vi "Run (lvsound2).vi"(8 "error in (no error)":errorcluster, 11 "Audio Output Queue":refnum<queue>) -> (0 "error out":errorcluster)   [LabVIEW 2019, in "Audio Output.lvlib"]
doc: "The main audio output loop.\n\n<b>Priority:</b> Time Critical\n<b>Execution System:</b> Instrument I/O"
uses:
  Audio Output.lvlib
  Audio Output Queue Type.ctl
  State.ctl
  Messaging/Message Cluster.ctl
  Audio Output Config.ctl
  Audio Output Info.ctl
  <vilib>/sound2/lvsound2.llb/Sound Data Format.ctl
  <vilib>/sound2/lvsound2.llb/Sound Output Task ID.ctl
  Globals/Constants.vi
  Globals/Debug.vi
  <vilib>/sound2/lvsound2.llb/Sound Output Write (I16).vi
  Messaging/Messaging.lvlib
  Globals/Globals.lvlib
  <vilib>/ptbypt/NI_PtbyPt.lvlib
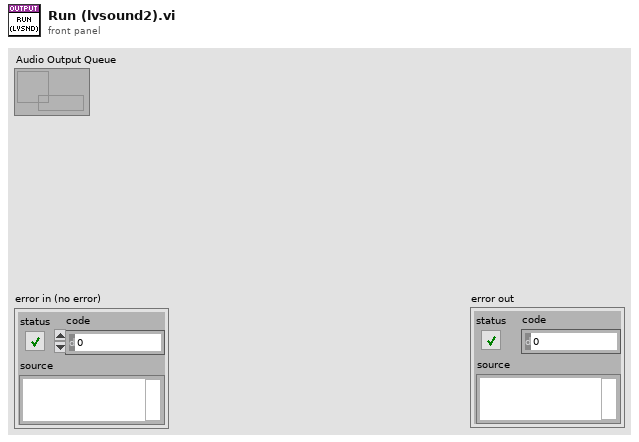
[diagram p1: front panel]
types:
  T1 = typedef "Audio Output.lvlib/Audio Output Config.ctl" = cluster{"Master":T2, "Headphones":T2}
  T2 = typedef "Audio Output.lvlib/Audio Output Info.ctl" = cluster{"Enable":bool, "Output ID":i32}
  T3 = typedef "Messaging.lvlib/Message Cluster.ctl" = cluster{"Event":string, "Source":string, "Target":string, "Data":variant}
  T4 = typedef "Audio Output.lvlib/State.ctl" = enum16{"Init", "Configure", "Output", "Error", "Shutdown"}
  T5 = typedef "Sound Data Format.ctl" = cluster{"sample rate (S/s)":dbl, "number of channels":i32, "bits per sample":i32}
  T6 = typedef "Sound Output Task ID.ctl" = u32
  T7 = typedef "Audio Output.lvlib/Audio Output Queue Type.ctl" = cluster{"Master":waveform(i16)[], "Headphones":waveform(i16)[], "Start Time":dbl}
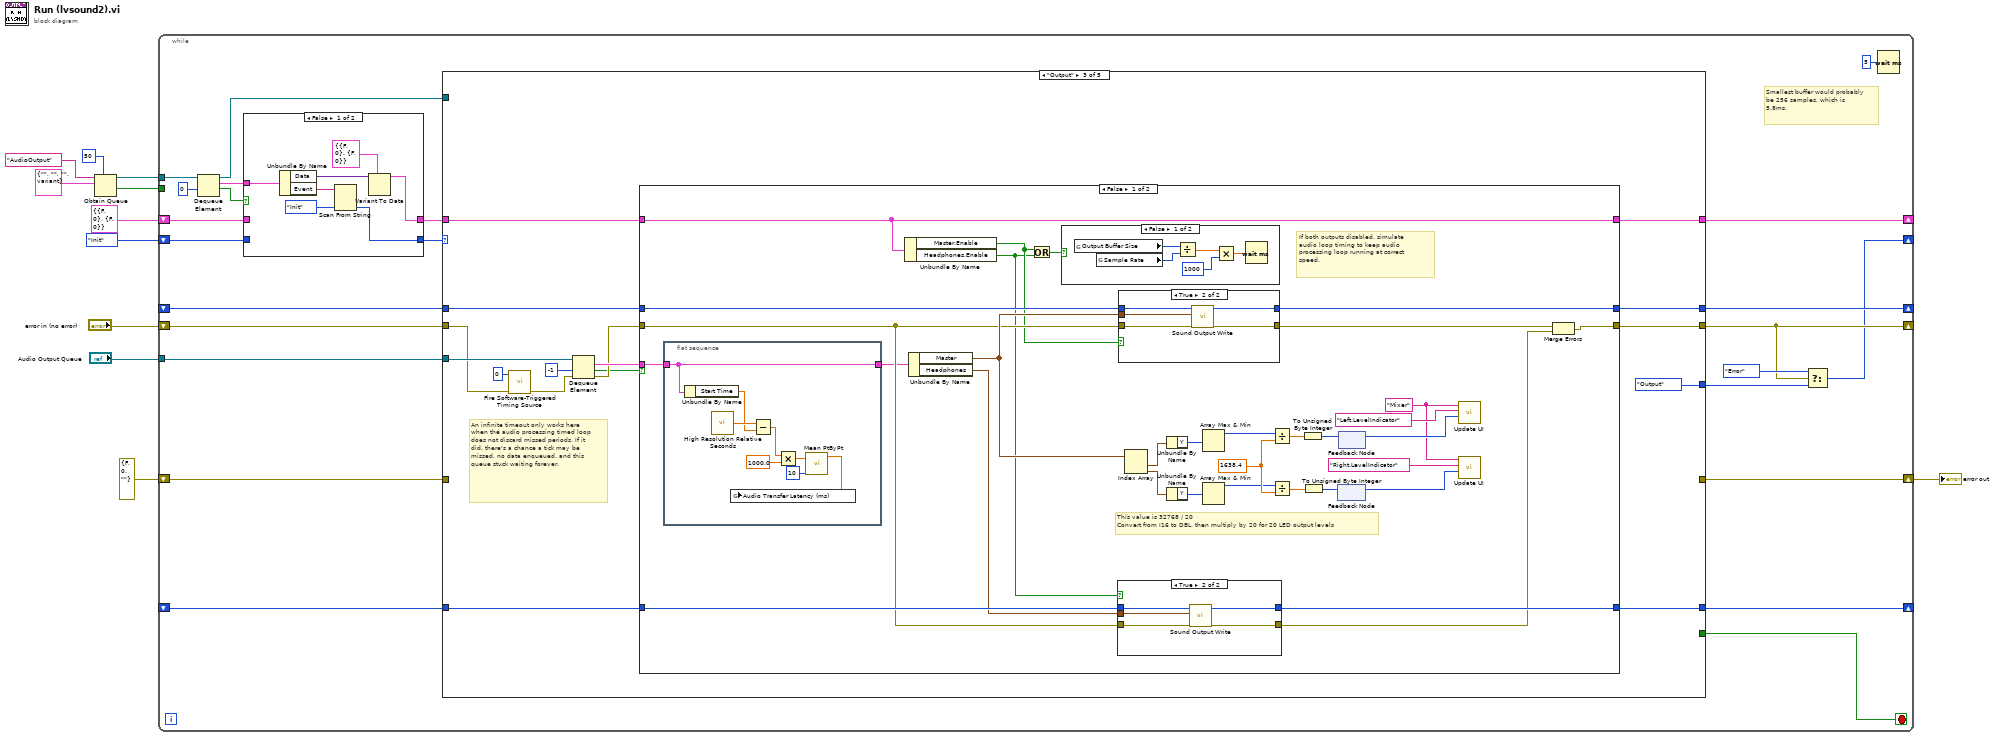
[diagram p0: block diagram]
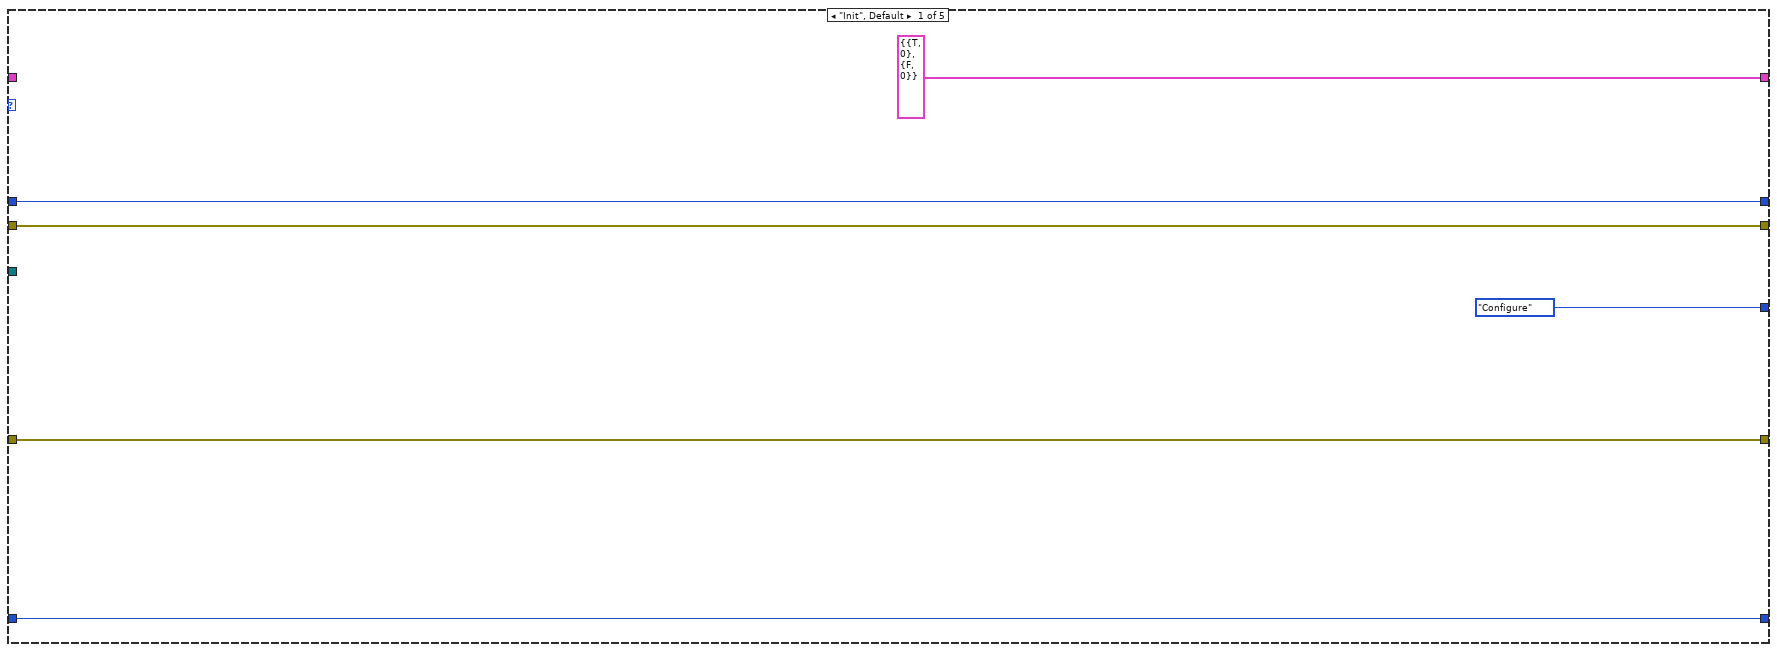
[diagram p3: hidden frame]
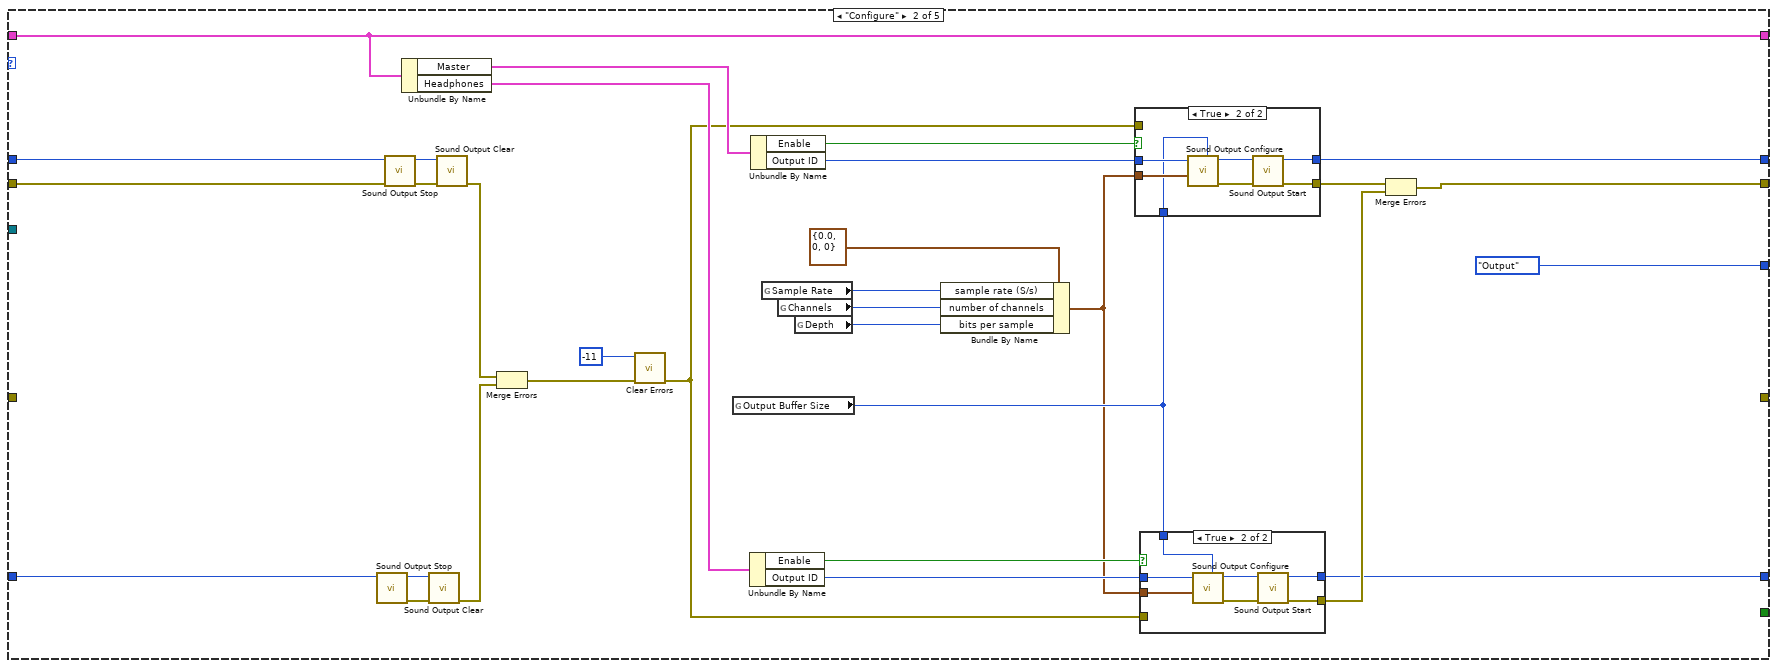
[diagram p4: hidden frame]
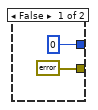
[diagram p5: hidden frame]
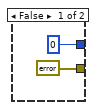
[diagram p6: hidden frame]
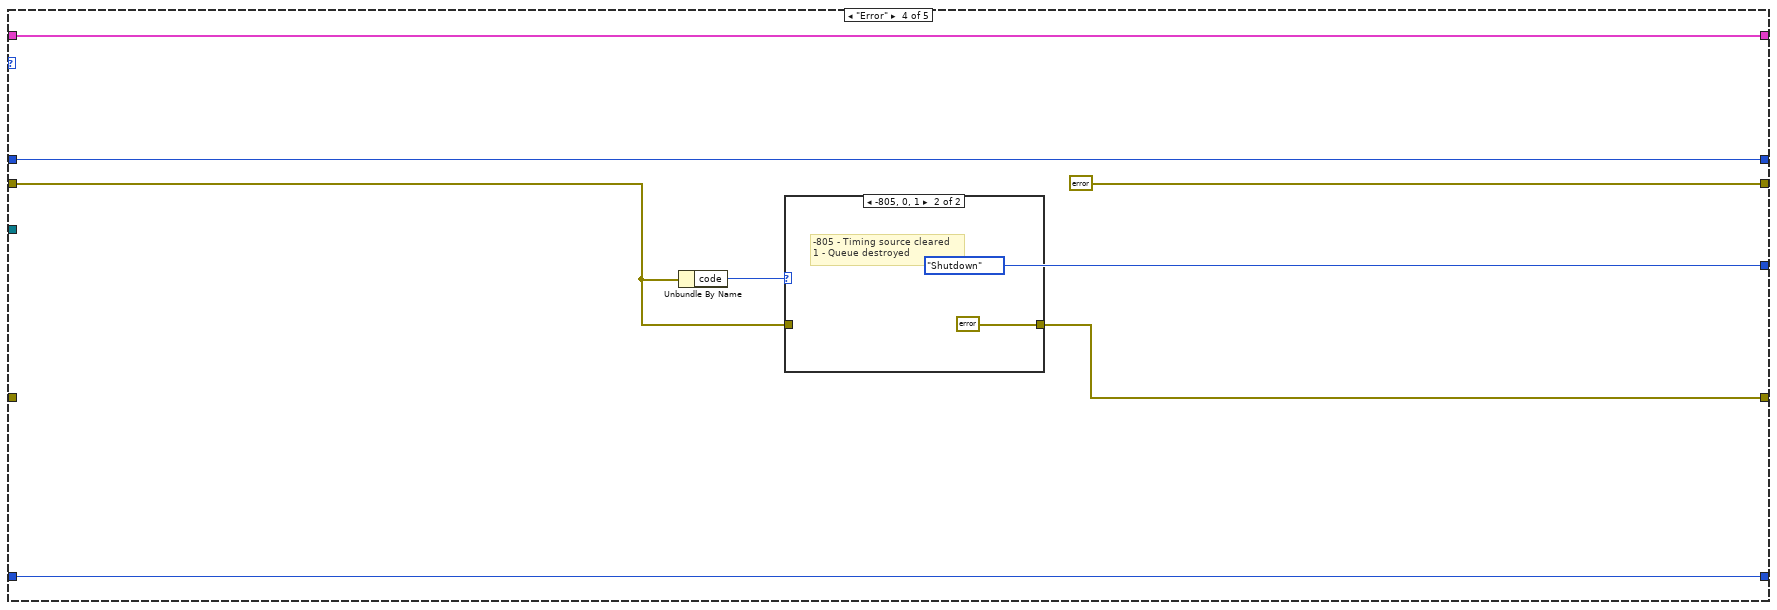
[diagram p11: hidden frame]
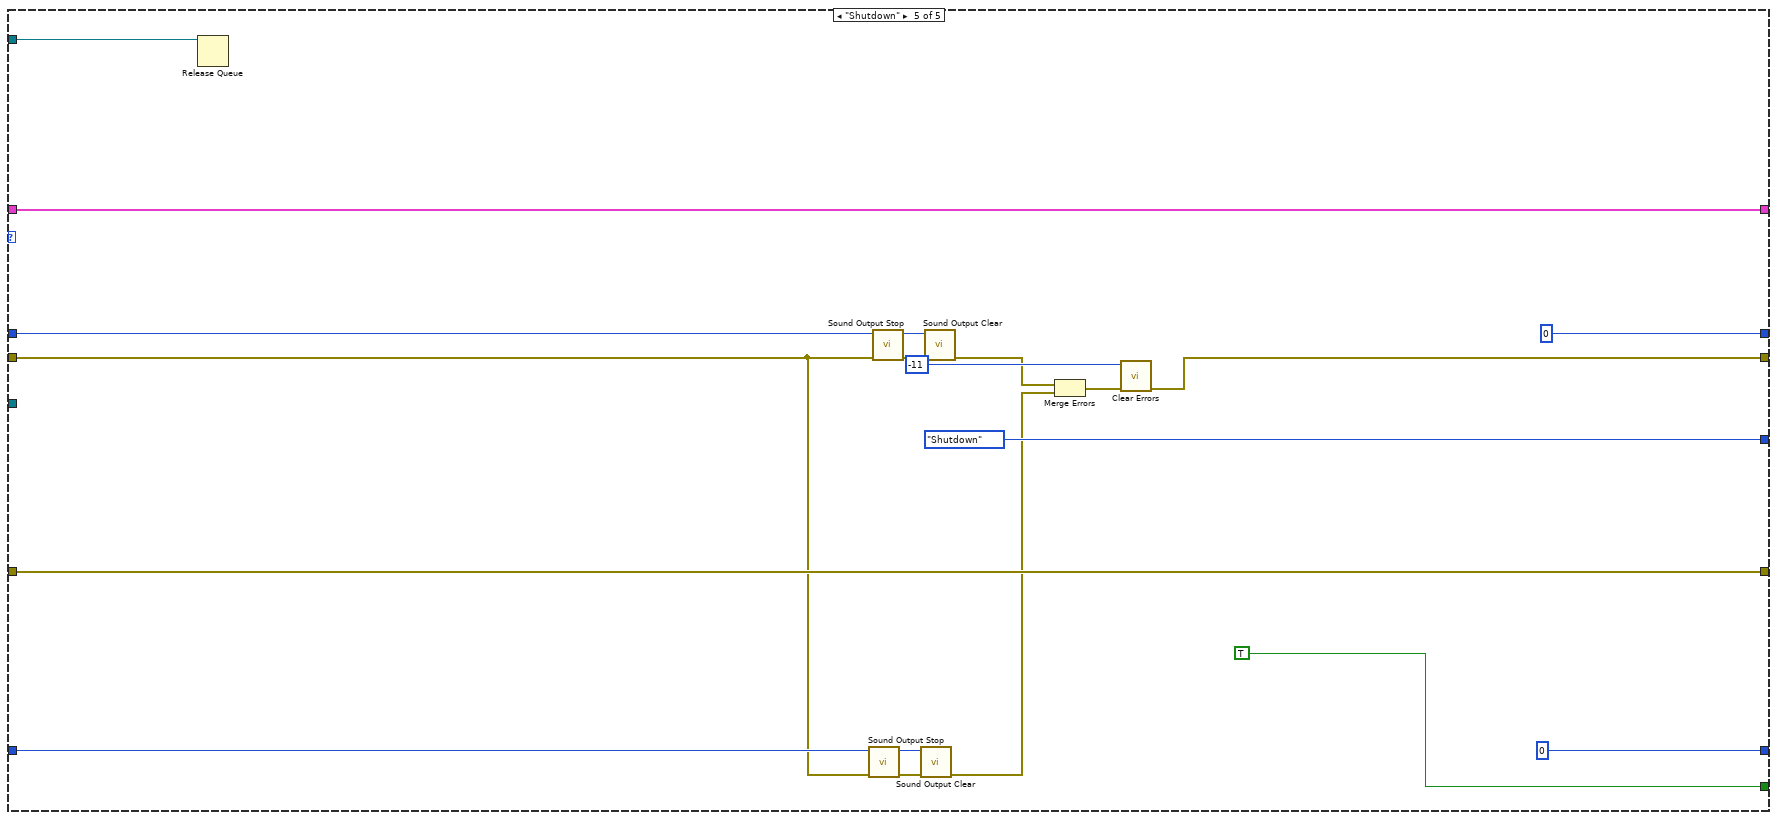
[diagram p13: hidden frame]
diagram:
  n1 = Obtain Queue(max queue size (-1, unlimited)=50, name (unnamed)="AudioOutput", element data type=T3 {"Event"="", "Source"="", "Target"="", "Data"=variant} ("Message")) -> (queue out=w4:refnum<queue>, created new?=w3:bool)  [unwired: 2 in, 1 out]
  n2 = while {
    shift-right: [w30] -> _
    shift-left: State."Init" ("State") -> [w18]
    shift-right: [w35] -> _
    shift-left: _ -> [w34]
    shift-right: [w31] -> _
    shift-left: "error in (no error)" -> [w28]
    tunnel: "Audio Output Queue" -> [w26]
    shift-right: [w25] -> w9
    shift-left: errorcluster {"status"=FALSE, "code"=0, "source"=""} ("error out") -> [w24]
    shift-right: [w23] -> _
    shift-left: _ -> [w22]
    tunnel: w4 -> [w20]
    shift-right: [w12] -> _
    shift-left: T1 {"Master"={"Enable"=FALSE, "Output ID"=0}, "Headphones"={"Enable"=FALSE, "Output ID"=0}} -> [w14]
    tunnel: w3 -> [_]
    stop <- w27 stop-if-true
    # "Smallest buffer would probably be 256 samples, which is 5.8ms."
    n3 = Dequeue Element(queue=w20, timeout in ms (-1)=0) -> (queue out=w15:refnum<queue>, element=w19:T3, timed out?=w16:bool)  [unwired: 1 in, 1 out]
    n4 = case shown="False" w16 {
      tunnel: w19 -> [w42 _]
      tunnel: w18 -> [_ w44]
      tunnel: [w39 w44] -> w17
      tunnel: [w36 w43] -> w13
      tunnel: w14 -> [_ w43]
      frame False {
        n5 = Unbundle By Name(w42) -> ("Data"=w37:variant, "Event"=w41:string)
        n6 = Scan From String(input string=w41, default 1=State."Init" ("State")) -> (output 1=w39:T4)  [unwired: 3 in, 3 out]
        n7 = Variant To Data(type=T1 {"Master"={"Enable"=FALSE, "Output ID"=0}, "Headphones"={"Enable"=FALSE, "Output ID"=0}}, Variant=w37) -> (data=w36:T1)  [unwired: 1 in, 1 out]
      }
      frame True {
      }
    }
    n8 = case shown="\"Output\"" w17 {
      tunnel: [w49 w81 w113 w186 T6 0 ("task ID out")] -> w35
      tunnel: w34 -> [w49 w66 w115 w186 w197]
      tunnel: [w48 w78 w114 errorcluster {"status"=FALSE, "code"=0, "source"=""} ("error out") w201] -> w31
      tunnel: [State."Configure" ("State") State."Output" ("State") State."Output" ("State") State."Shutdown" ("State") State."Shutdown" ("State")] -> w33
      tunnel: w28 -> [w48 w63 w101 w182 w192]
      tunnel: [_ _ _ _ TRUE] -> w27
      tunnel: w26 -> [_ _ w109 _ _]
      tunnel: [w47 _ _ w181 w205] -> w25
      tunnel: w24 -> [w47 _ _ _ w205]
      tunnel: [w46 w57 w106 w180 T6 0 ("task ID out")] -> w23
      tunnel: w22 -> [w46 w59 w105 w180 w193]
      tunnel: w15 -> [_ _ _ _ w204]
      tunnel: w13 -> [_ w73 w103 w179 w203]
      tunnel: [T1 {"Master"={"Enable"=TRUE, "Output ID"=0}, "Headphones"={"Enable"=FALSE, "Output ID"=0}} ("Audio Output Config") w73 w104 w179 w203] -> w12
      frame "Init", Default {
      }
      frame "Configure" {
        n9 = call <vilib>:"Sound Output Stop.vi"("task ID"=w59) -> ("error out"=w61:errorcluster, "task ID out"=w60:T6)  [unwired: 9 in]
        n10 = call <vilib>:"Sound Output Stop.vi"("error in (no error)"=w63, "task ID"=w66) -> ("error out"=w64:errorcluster, "task ID out"=w65:T6)  [unwired: 8 in]
        n11 = Unbundle By Name(w73) -> ("Master"=w77:T2, "Headphones"=w74:T2)
        n12 = call <vilib>:"Sound Output Clear.vi"("error in (no error)"=w61, "task ID"=w60) -> ("error out"=w58:errorcluster)  [unwired: 9 in]
        n13 = call <vilib>:"Sound Output Clear.vi"("error in (no error)"=w64, "task ID"=w65) -> ("error out"=w62:errorcluster)  [unwired: 9 in]
        n14 = Merge Errors(w62, w58) -> (w72:errorcluster)
        n15 = call <vilib>:"Clear Errors.vi"("error in (no error)"=w72, "specific error code to clear (0: all)"=-11) -> ("error out"=w67:errorcluster)  [unwired: 4 in, 1 out]
        n16 = global read "Constants.vi" "Output Buffer Size"() -> (w52:i32)
        n17 = Unbundle By Name(w74) -> ("Enable"=w70:bool, "Output ID"=w69:i32)
        n18 = Unbundle By Name(w77) -> ("Enable"=w71:bool, "Output ID"=w75:i32)
        n19 = global read "Constants.vi" "Sample Rate"() -> (w55:i32)
        n20 = global read "Constants.vi" "Channels"() -> (w54:i32)
        n21 = global read "Constants.vi" "Depth"() -> (w53:i32)
        n22 = Bundle By Name(cluster=T5 {"sample rate (S/s)"=0.0, "number of channels"=0, "bits per sample"=0} ("sound format"), "sample rate (S/s)"=w55, "number of channels"=w54, "bits per sample"=w53) -> (w51:T5)
        n23 = case shown="True" w71 {
          tunnel: [T6 0 ("task ID out") w99] -> w81
          tunnel: [errorcluster {"status"=FALSE, "code"=0, "source"=""} ("error out") w94] -> w79
          tunnel: w75 -> [_ w96]
          tunnel: w67 -> [_ _]
          tunnel: w51 -> [_ w97]
          tunnel: w52 -> [_ w95]
          frame False {
          }
          frame True {
            n24 = call <vilib>:"Sound Output Configure.vi"("number of samples/ch"=w95, "sound format"=w97, "device ID"=w96) -> ("error out"=w93:errorcluster, "task ID"=w98:T6)  [unwired: 7 in]
            n25 = call <vilib>:"Sound Output Start.vi"("error in (no error)"=w93, "task ID"=w98) -> ("error out"=w94:errorcluster, "task ID out"=w99:T6)  [unwired: 8 in]
          }
        }
        n26 = case shown="True" w70 {
          tunnel: [T6 0 ("task ID out") w90] -> w57
          tunnel: [errorcluster {"status"=FALSE, "code"=0, "source"=""} ("error out") w86] -> w68
          tunnel: w69 -> [_ w87]
          tunnel: w51 -> [_ w88]
          tunnel: w67 -> [_ _]
          tunnel: w52 -> [_ w85]
          frame False {
          }
          frame True {
            n27 = call <vilib>:"Sound Output Configure.vi"("number of samples/ch"=w85, "sound format"=w88, "device ID"=w87) -> ("error out"=w84:errorcluster, "task ID"=w89:T6)  [unwired: 7 in]
            n28 = call <vilib>:"Sound Output Start.vi"("error in (no error)"=w84, "task ID"=w89) -> ("error out"=w86:errorcluster, "task ID out"=w90:T6)  [unwired: 8 in]
          }
        }
        n29 = Merge Errors(w79, w68) -> (w78:errorcluster)
      }
      frame "Output" {
        # "An infinite timeout only works here when the audio processing timed loop does not discard missed periods. If it did, there's a chance a tick may be missed, no data enqueued, and this queue stuck waiting forever."
        n30 = call <vilib>:"Fire Software-Triggered Timing Source.vi"("error in (no error)"=w101, "trigger ID"=u8 0) -> ("error out"=w102:errorcluster)  [unwired: 8 in, 1 out]
        n31 = Dequeue Element(queue=w109, timeout in ms (-1)=-1, error in (no error)=w102) -> (element=w111:T7, timed out?=w107:bool, error out=w108:errorcluster)  [unwired: 1 out]
        n32 = case shown="False" w107 {
          tunnel: w115 -> [w136 w178]
          tunnel: [w130 w177] -> w114
          tunnel: [w135 w178] -> w113
          tunnel: w111 -> [w117 _]
          tunnel: w108 -> [w126 w177]
          tunnel: [w134 w176] -> w106
          tunnel: w105 -> [w133 w176]
          tunnel: [w127 w175] -> w104
          tunnel: w103 -> [w127 w175]
          frame False {
            w120 = "Mixer" ("ID")
            w143 = 1638.4
            # "If both outputs disabled, simulate audio loop timing to keep audio processing loop running at correct speed."
            # "This value is 32768 / 20\nConvert from I16 to DBL, then multiply by 20 for 20 LED output levels"
            n33 = flat-sequence {
              tunnel: w117 -> [w155]
              tunnel: [w155] -> w116
              frame #0 {
                n34 = Unbundle By Name(w155) -> ("Start Time"=w153:dbl)
                n35 = call <vilib>:"High Resolution Relative Seconds.vi"() -> ("relative seconds"=w154:dbl)
                n36 = Subtract(x=w154, y=w153) -> (x-y=w152:dbl)
                n37 = Multiply(x=w152, y=1000.0) -> (x*y=w150:dbl)
                n38 = call <vilib>:"Mean PtByPt.vi"("x"=w150, "sample length"=10) -> ("mean"=w149:dbl)  [unwired: 2 in, 1 out]
                n39 = global write "Debug.vi" "Audio Transfer Latency (ms)"(w149) -> ()
              }
            }
            n40 = Unbundle By Name(w127) -> ("Master.Enable"=w125:bool, "Headphones.Enable"=w124:bool)
            n41 = Unbundle By Name(w116) -> ("Master"=w129:waveform(i16)[], "Headphones"=w128:waveform(i16)[])
            n42 = Or(x=w125, y=w124) -> (x .or. y?=w123:bool)
            n43 = case shown="False" w123 {
              frame False {
                n44 = global read "Constants.vi" "Output Buffer Size"() -> (w156:i32)
                n45 = global read "Constants.vi" "Sample Rate"() -> (w157:i32)
                n46 = Divide(x=w156, y=w157) -> (x/y=w159:dbl)
                n47 = Multiply(x=w159, y=1000) -> (x*y=w158:dbl)
                n48 = Wait (ms)(milliseconds to wait=w158) -> ()  [unwired: 1 out]
              }
              frame True {
              }
            }
            n49 = case shown="True" w124 {
              tunnel: [w162 w165] -> w134
              tunnel: w133 -> [w162 w167]
              tunnel: [w161 w163] -> w132
              tunnel: w128 -> [_ w166]
              tunnel: w126 -> [w161 w164]
              frame False {
              }
              frame True {
                n50 = call-poly <vilib>:"Sound Output Write.vi"("error in (no error)"=w164, "data"=w166, "task ID"=w167) -> ("error out"=w163:errorcluster, "task ID out"=w165:T6)  [unwired: 7 in]
              }
            }
            n51 = case shown="True" w125 {
              tunnel: w136 -> [w169 w174]
              tunnel: [w169 w173] -> w135
              tunnel: w126 -> [w168 w172]
              tunnel: [w168 w171] -> w131
              tunnel: w129 -> [_ w170]
              frame False {
              }
              frame True {
                n52 = call-poly <vilib>:"Sound Output Write.vi"("error in (no error)"=w172, "data"=w170, "task ID"=w174) -> ("error out"=w171:errorcluster, "task ID out"=w173:T6)  [unwired: 7 in]
              }
            }
            n53 = Index Array(array=w129) -> (element #1=w138:waveform(i16), element #2=w139:waveform(i16))  [unwired: 2 in]
            n54 = Unbundle By Name(w138) -> ("Y"=w137:i16[])
            n55 = Unbundle By Name(w139) -> ("Y"=w140:i16[])
            n56 = Array Max & Min(array=w137) -> (max value=w141:i16)  [unwired: 3 out]
            n57 = Array Max & Min(array=w140) -> (max value=w142:i16)  [unwired: 3 out]
            n58 = Divide(x=w141, y=w143) -> (x/y=w144:dbl)
            n59 = Divide(x=w142, y=w143) -> (x/y=w145:dbl)
            n60 = To Unsigned Byte Integer(number=w144) -> (unsigned 8bit integer=w146:u8)
            n61 = To Unsigned Byte Integer(number=w145) -> (unsigned 8bit integer=w147:u8)
            n62 = feedback #1() -> (w118:u8)  [unwired: 1 in]
            n63 = feedback-in #1(w147) -> ()
            n64 = feedback #2() -> (w121:u8)  [unwired: 1 in]
            n65 = feedback-in #2(w146) -> ()
            n66 = call "Update UI.vi"("Data"=w121, "Target"="Left.LevelIndicator", "ID"=w120) -> ()  [unwired: 8 in, 1 out]
            n67 = call "Update UI.vi"("Data"=w118, "Target"="Right.LevelIndicator", "ID"=w120) -> ()  [unwired: 8 in, 1 out]
            n68 = Merge Errors(w131, w132) -> (w130:errorcluster)
          }
          frame True {
          }
        }
      }
      frame "Error" {
        n69 = Unbundle By Name(w182) -> ("code"=w183:i32)
        n70 = case shown="-805, 0, 1" w183 {
          tunnel: w182 -> [w187 _]
          tunnel: [w187 errorcluster {"status"=FALSE, "code"=0, "source"=""} ("error out")] -> w181
          frame Default {
          }
          frame -805, 0, 1 {
            # "-805 - Timing source cleared\n1 - Queue destroyed"
          }
        }
      }
      frame "Shutdown" {
        n71 = Release Queue(queue=w204) -> ()  [unwired: 2 in, 3 out]
        n72 = call <vilib>:"Sound Output Stop.vi"("error in (no error)"=w192, "task ID"=w193) -> ("error out"=w195:errorcluster, "task ID out"=w194:T6)  [unwired: 8 in]
        n73 = call <vilib>:"Sound Output Stop.vi"("error in (no error)"=w192, "task ID"=w197) -> ("error out"=w198:errorcluster, "task ID out"=w199:T6)  [unwired: 8 in]
        n74 = call <vilib>:"Sound Output Clear.vi"("error in (no error)"=w195, "task ID"=w194) -> ("error out"=w191:errorcluster)  [unwired: 9 in]
        n75 = call <vilib>:"Sound Output Clear.vi"("error in (no error)"=w198, "task ID"=w199) -> ("error out"=w196:errorcluster)  [unwired: 9 in]
        n76 = Merge Errors(w196, w191) -> (w202:errorcluster)
        n77 = call <vilib>:"Clear Errors.vi"("error in (no error)"=w202, "specific error code to clear (0: all)"=-11) -> ("error out"=w201:errorcluster)  [unwired: 4 in, 1 out]
      }
    }
    n78 = Select(t=State."Error" ("State"), s=w31, f=w33) -> (s? t:f=w30:T4)
    n79 = Wait (ms)(milliseconds to wait=u32 5 ("millisecond multiple")) -> ()  [unwired: 1 out]
  }
  "error out" <- w9
